vi "DN4_DDT22Darray.vi"(1 "data":dynamicdata(waveform)) -> (0 "Array":dbl[][](array[numeric]))   [LabVIEW 2009]
uses:
  Instance           1 19Saved   DDT22Darray .vi
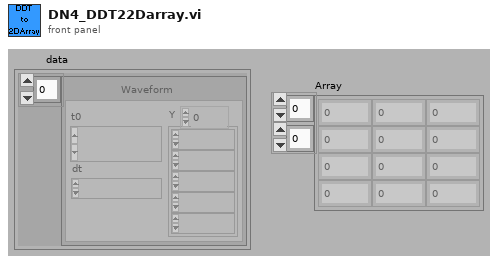
[diagram p1: front panel]
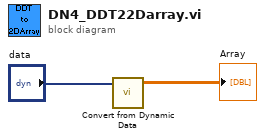
[diagram p0: block diagram]
diagram:
  n1 = call "Convert from Dynamic Data"("Dynamic Data Type"="data") -> ("Array"=→"Array":dbl[][])  [unwired: 3 out]
